vi "Status Current Status.vi"(5 "Retry Attempts (0)":i32 min=0, 8 "error in (no error)":errorcluster, 11 "VISA resource name":refnum<visa-resource-name>) -> (0 "error out":errorcluster, 2 "Status Cluster":T1, 3 "VISA resource name out":refnum<visa-resource-name>)   [LabVIEW 2020, in "ChromTech Series III Pump.lvlib"]
doc: "Returns the current flow rate* in ml/min, upper pressure limit, lower pressure limit, pressure units, and the run/stop state, where True = running and False = stopped.\n\n*CP pumps return flow rate set point"
uses:
  <instrlib>/ChromTech Series III Pump/ChromTech Series III Pump.lvlib
panel:
  out "Response":string
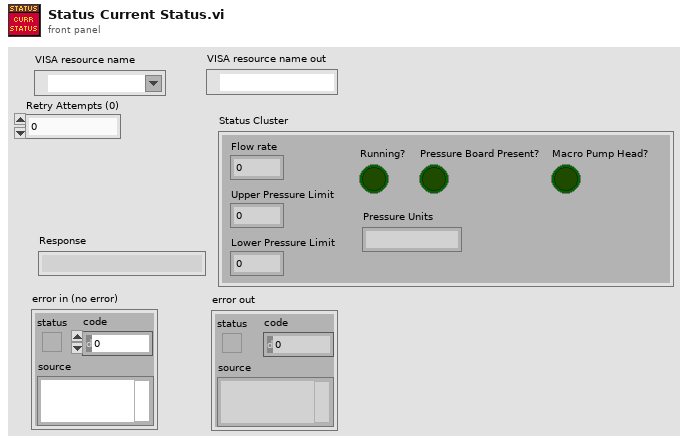
[diagram p1: front panel]
types:
  T1 = cluster{"Flow rate":dbl, "Upper Pressure Limit":dbl, "Lower Pressure Limit":dbl, "Pressure Units":string, "Running?":bool, "Pressure Board Present?":bool, "Macro Pump Head?":bool}
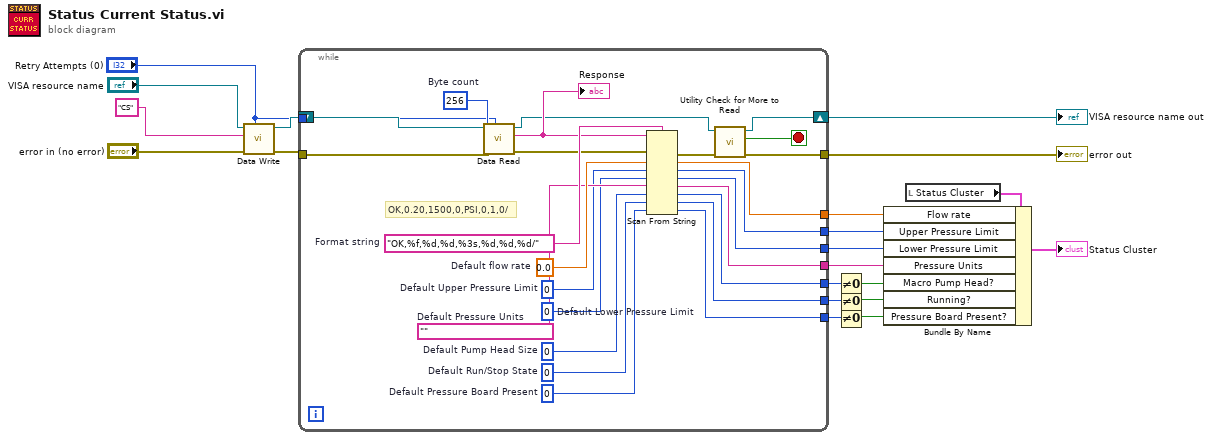
[diagram p0: block diagram]
diagram:
  n1 = call <instrlib>:"Data Write.vi"("Retry Attempts (0)"="Retry Attempts (0)", "error in (no error)"="error in (no error)", "Command"="CS" ("command"), "VISA Refnum in"="VISA resource name") -> ("error out"=w3:errorcluster, "VISA Refnum out"=w2:refnum<visa-resource-name>)  [unwired: 6 in]
  n2 = while {
    tunnel: [w44] -> w17
    tunnel: [w43] -> w14
    tunnel: [w42] -> w13
    tunnel: [w41] -> w12
    tunnel: [w40] -> w11
    tunnel: [w31] -> w5
    tunnel: [w30] -> w4
    tunnel: "Retry Attempts (0)" -> [w26]
    shift-right: [w23] -> w18
    shift-left: w2 -> [w27]
    tunnel: w3 -> [w29]
    tunnel: [w22] -> w9
    stop <- w21 stop-if-true
    w28 = u32 256  # Byte count
    w32 = 0  # Default Pressure Board Present
    w34 = 0  # Default Pump Head Size
    w36 = 0  # Default Lower Pressure Limit
    w37 = 0  # Default Upper Pressure Limit
    w33 = 0  # Default Run/Stop State
    w38 = ""  # Default Pressure Units
    w39 = 0.0  # Default flow rate
    w46 = "OK,%f,%d,%d,%3s,%d,%d,%d/"  # Format string
    # "OK,0.20,1500,0,PSI,0,1,0/"
    n3 = call <instrlib>:"Data Read.vi"("Retry Attempts (0)"=w26, "error in (no error)"=w29, "Bytes to read"=w28, "VISA Refnum in"=w27) -> ("error out"=w45:errorcluster, "read buffer"=w35:string, "VISA Refnum out"=w24:refnum<visa-resource-name>)  [unwired: 5 in]
    "Response" <- w35
    n4 = Scan From String(format string=w46, input string=w35, error in=w45, default 1=w39, default 2=w37, default 3=w36, default 4=w38, default 5=w34, default 6=w33, default 7=w32) -> (error out=w25:errorcluster, output 1=w40:dbl, output 2=w41:i32, output 3=w42:i32, output 4=w43:string, output 5=w44:i32, output 6=w31:i32, output 7=w30:i32)  [unwired: 1 in, 2 out]
    n5 = call <instrlib>:"Utility Check for More to Read.vi"("error in (no error)"=w25, "VISA Refnum in"=w24) -> ("error out (unchanged)"=w22:errorcluster, "More to read?"=w21:bool, "VISA Refnum out"=w23:refnum<visa-resource-name>)  [unwired: 7 in]
  }
  "VISA resource name out" <- w18
  "error out" <- w9
  n6 = Not Equal To 0?(x=w17) -> (x != 0?=w15:bool)
  n7 = Not Equal To 0?(x=w5) -> (x != 0?=w7:bool)
  n8 = Not Equal To 0?(x=w4) -> (x != 0?=w6:bool)
  n9 = local read "Status Cluster"() -> (w16:T1)
  n10 = Bundle By Name(cluster=w16, "Flow rate"=w11, "Upper Pressure Limit"=w12, "Lower Pressure Limit"=w13, "Pressure Units"=w14, "Macro Pump Head?"=w15, "Running?"=w7, "Pressure Board Present?"=w6) -> (→"Status Cluster":T1)
